vi "Neopixel-Globals.vi"() -> ()   [LabVIEW 2020]
panel:
  in  "Version":string
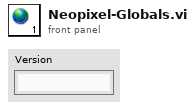
[diagram p1: front panel]
diagram:
